vi "Init.vi"(8 "error in (no error)":errorcluster, 10 "IConfigure in":refnum<class "IConfigure.lvclass">, 11 "Thermometer Base in":refnum<class "Thermometer Base.lvclass">) -> (0 "error out":errorcluster, 3 "Thermometer Base out":refnum<class "Thermometer Base.lvclass">)   [LabVIEW 2023, in "Thermometer.lvlib" / "Thermometer Base.lvlib" / "Thermometer Base.lvclass"]
uses:
  Thermometer Base.lvclass
  Interfaces/IConfigure/IConfigure.lvclass
  Thermometer Base.lvclass/Thermometer Base.ctl
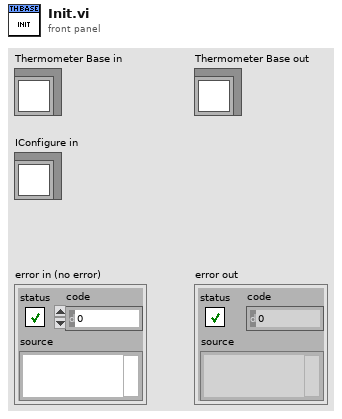
[diagram p1: front panel]
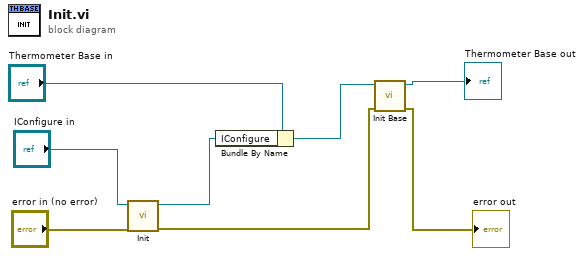
[diagram p0: block diagram]
diagram:
  n1 = call-dynamic "Init.vi"("error in"="error in (no error)", "IConfigure in"="IConfigure in") -> ("error out"=w7:errorcluster, "IConfigure out"=w8:refnum<class "IConfigure.lvclass">)  [unwired: 8 in]
  n2 = Bundle By Name(cluster="Thermometer Base in", "IConfigure"=w8) -> (w6:refnum<class "Thermometer Base.lvclass">)
  n3 = call-dynamic "Init Base.vi"("Error In"=w7, "object in"=w6) -> ("Error Out"=→"error out":errorcluster, "object out"=→"Thermometer Base out":refnum<class "Thermometer Base.lvclass">)  [unwired: 8 in]
